vi "Do.vi"(8 "error in (no error)":cluster{"状态":bool, "代码":i32, "源":string} caption="错误输入（无错误）", 10 "操作者输入":refnum<class "Actor.lvclass">, 11 "Task B任务消息":refnum<class "Task B任务消息.lvclass">) -> (0 "error out":cluster{"状态":bool, "代码":i32, "源":string} caption="错误输出", 2 "操作者输出":refnum<class "Actor.lvclass">)   [LabVIEW 2013, in "Task B操作者.lvlib" / "Task B任务消息.lvclass"]
uses:
  <vilib>/ActorFramework/Actor/Actor.lvclass
  Task B/Task B.lvclass
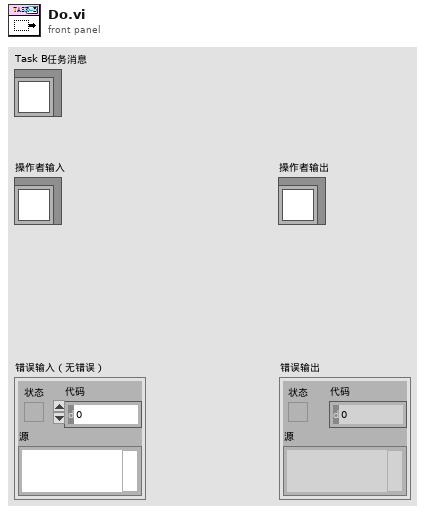
[diagram p1: front panel]
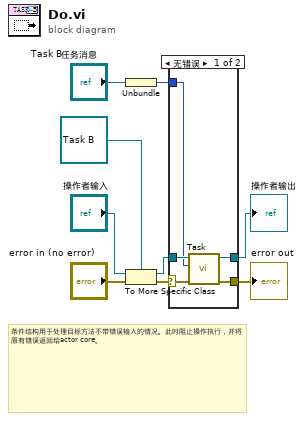
[diagram p0: block diagram]
diagram:
  # "条件结构用于处理目标方法不带错误输入的情况。此时阻止操作执行，并将原有错误返回给actor core。"
  n1 = Unbundle("Task B任务消息") -> (w1:i32)
  n2 = To More Specific Class(target class=refnum<class "Task B.lvclass"> refnum ("Actor in"), reference="操作者输入", error in="error in (no error)") -> (specific class reference=w8:refnum<class "Task B.lvclass">, error out=w4:errorcluster)
  n3 = case shown="无错误" w4 {
    selector: w4 -> [w11 w16]
    tunnel: w8 -> [w14 w15]
    tunnel: [w13 w16] -> w3
    tunnel: [w12 w15] -> w2
    tunnel: w1 -> [w10 _]
    frame No Error {
      n4 = call-dynamic "Task.vi"("error in (no error)"=w11, "数据"=w10, "Task B输入"=w14) -> ("error out"=w13:cluster{"状态":bool, "代码":i32, "源":string}, "Task B输出"=w12:refnum<class "Task B.lvclass">)  [unwired: 7 in]
    }
    frame Error {
    }
  }
  "error out" <- w3
  "操作者输出" <- w2
